vi "Q10_transfer_2_X.vi"(3 "Qn":dbl[](array[numeric]), 4 "x":dbl format="%#_13g") -> (1 "y":dbl)   [LabVIEW 2015]
panel:
  out "x*y 2":dbl[](array[numeric])
  out "xk chain":dbl[](array[numeric])
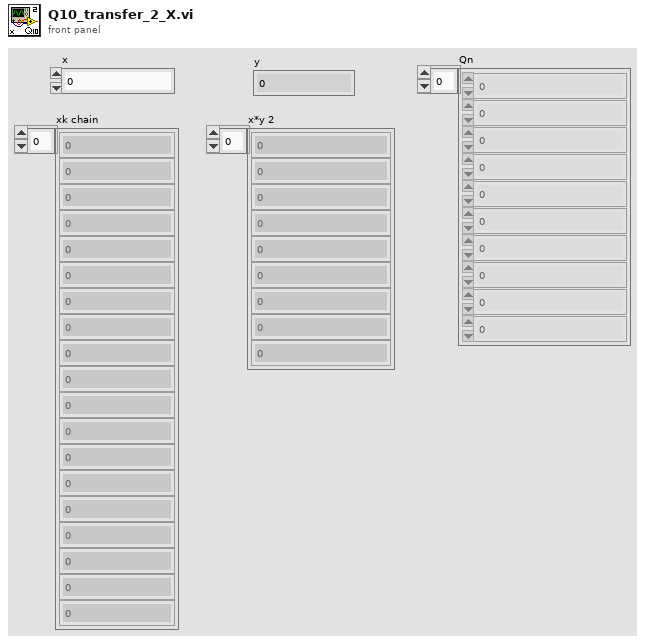
[diagram p1: front panel]
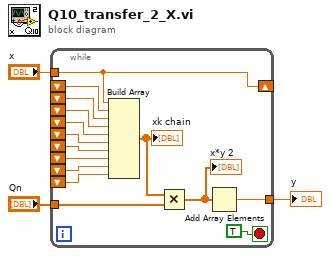
[diagram p0: block diagram]
diagram:
  n1 = while {
    tunnel: [w9] -> w3
    tunnel: "x" -> [w17]
    tunnel: "Qn" -> [w13]
    shift-right: [w17] -> _
    shift-left: _ -> [w16]
    shift-left: _ -> [w12]
    shift-left: _ -> [w11]
    shift-left: _ -> [w10]
    shift-left: _ -> [w8]
    shift-left: _ -> [w7]
    shift-left: _ -> [w6]
    shift-left: _ -> [w5]
    shift-left: _ -> [w4]
    stop <- TRUE stop-if-true
    n2 = Build Array(w17, w16, w12, w11, w10, w8, w7, w6, w5, w4) -> (w14:dbl[])
    "xk chain" <- w14
    n3 = Multiply(x=w14, y=w13) -> (x*y=w18:dbl[])
    "x*y 2" <- w18
    n4 = Add Array Elements(numeric array=w18) -> (sum=w9:dbl)
  }
  "y" <- w3
